vi "StanfordResSysDG645DelayGeneratorToDLAY.vi"(9 "Control Array":refnum<vi>[](array[refnum]), 10 "Changed Names in":string[](array[string])) -> ()   [LabVIEW 2020]
uses:
  <vilib>/regexp/Match Regular Expression.xnode
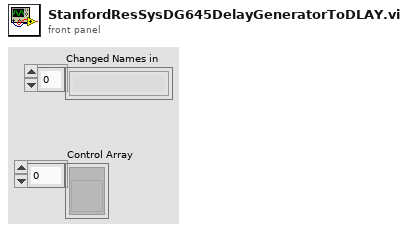
[diagram p1: front panel]
types:
  T1 = cluster{"[0]":string, "[1]":string, "[2]":string}
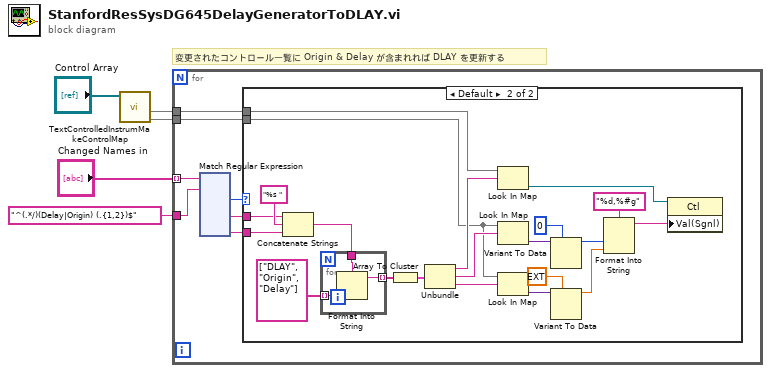
[diagram p0: block diagram]
diagram:
  # "変更されたコントロール一覧に Origin & Delay が含まれれば DLAY を更新する"
  n1 = call "TextControlledInstrumMakeControlMap.vi"("ControlArray"="Control Array") -> ("ValueMap out"=w3:map{string, variant}, "ControlMap out"=w2:map{string, refnum<vi>})  [unwired: 7 in, 2 out]
  n2 = for {
    tunnel: "Changed Names in" -> [w12] mode=indexing
    tunnel: "^(.*/)(Delay|Origin) (.{1,2})$" ("regular expression") -> [w11]
    tunnel: w3 -> [w10]
    tunnel: w2 -> [w7]
    n3 = xnode "Match Regular Expression"("input string"=w12, "regular expression"=w11) -> ("offset past match"=w6:i32, "submatch 1"=w9:string, "submatch 3"=w8:string)  [unwired: 4 in, 5 out]
    n4 = case shown="Default" w6 {
      tunnel: w10 -> [_ w13]
      tunnel: w9 -> [_ w25]
      tunnel: w8 -> [_ w24]
      tunnel: w7 -> [_ w23]
      frame -1 {
      }
      frame Default {
        n5 = Concatenate Strings(w25, "%s ", w24) -> (w21:string)
        n6 = for {
          tunnel: string[] ["DLAY", "Origin", "Delay"] -> [w36] mode=indexing
          tunnel: w21 -> [w35]
          tunnel: [w34] -> w20 mode=indexing
          n7 = Format Into String(format string=w35, w36) -> (resulting string=w34:string)  [unwired: 2 in, 1 out]
        }
        n8 = Array To Cluster(array=w20) -> (cluster=w19:T1)
        n9 = Unbundle(w19) -> ("[0]"=w15:string, "[1]"=w18:string, "[2]"=w14:string)
        n10 = Look In Map(map=w23, key=w15) -> (value=w17:refnum<vi>)  [unwired: 1 in, 1 out]
        n11 = Look In Map(map=w13, key=w18) -> (value=w32:variant)  [unwired: 1 in, 1 out]
        n12 = Look In Map(map=w13, key=w14) -> (value=w31:variant)  [unwired: 1 in, 1 out]
        n13 = Variant To Data(type=u32 0, Variant=w32) -> (data=w27:u32)  [unwired: 1 in, 1 out]
        n14 = Variant To Data(type=ext 0.0, Variant=w31) -> (data=w26:ext)  [unwired: 1 in, 1 out]
        n15 = Format Into String(format string="%d,%#g", w27, w26) -> (resulting string=w16:string)  [unwired: 2 in, 1 out]
        n16 = property class="Ctl"(reference=w17, "Val(Sgnl)"=w16) -> ()  [unwired: 1 in, 2 out]
      }
    }
  }
